vi "SRV_PM_VIG_Packet Mode.vi"(7 "Packet Mode Style":T1, 12 "Method (Get)":enum16{"Get", "Set"}(ring)) -> (8 "Packet Mode Style":T1)   [LabVIEW 2014]
uses:
  SRV_PM_Packet Mode Style.ctl
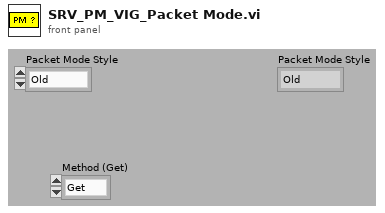
[diagram p1: front panel]
types:
  T1 = typedef "SRV_PM_Packet Mode Style.ctl" = enum16{"Old", "New PM"}
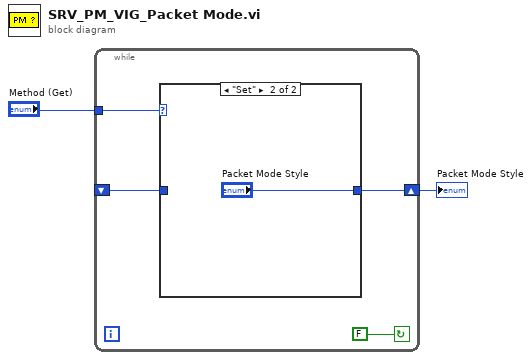
[diagram p0: block diagram]
diagram:
  n1 = while {
    shift-right: [w4] -> w1
    shift-left: _ -> [w3]
    tunnel: "Method (Get)" -> [w5]
    stop <- FALSE continue-if-true
    n2 = case shown="\"Set\"" w5 {
      tunnel: [w7 "Packet Mode Style"] -> w4
      tunnel: w3 -> [w7 _]
      frame "Get" {
      }
      frame "Set" {
      }
    }
  }
  "Packet Mode Style" <- w1
